vi "数据整合分析.vi"(10 "原始数据库":string[][](table), 11 "Data Result":string[][](table)) -> (3 "原始数据库 2":string[][](table))   [LabVIEW 2015]
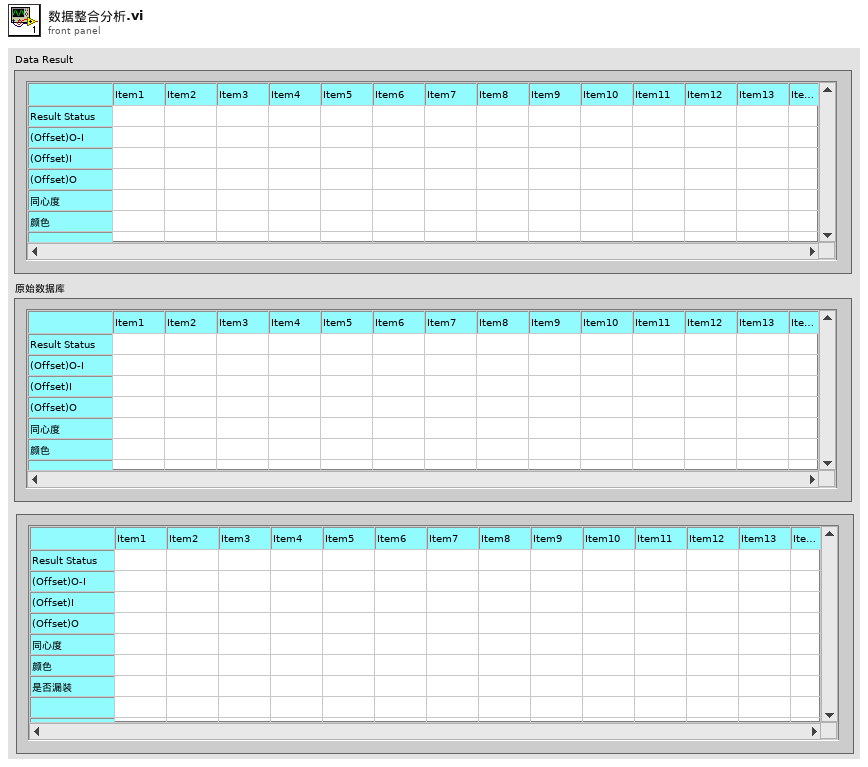
[diagram p1: front panel]
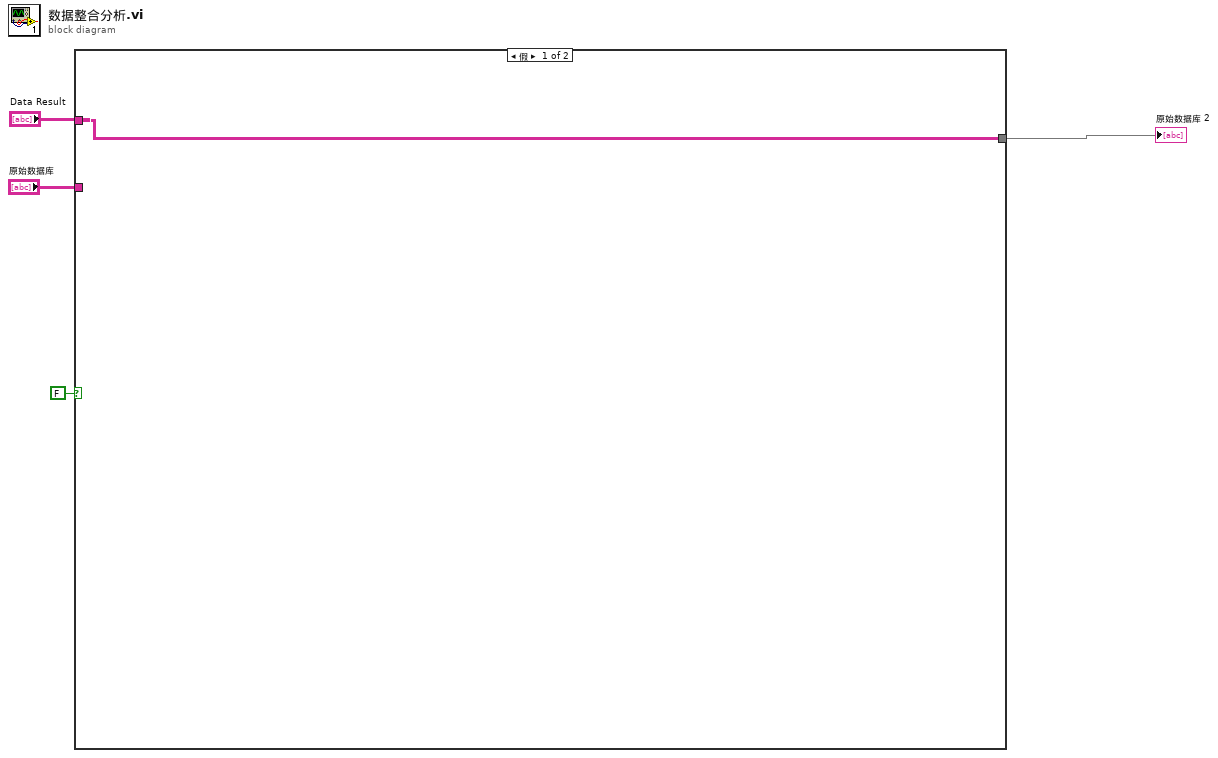
[diagram p0: block diagram]
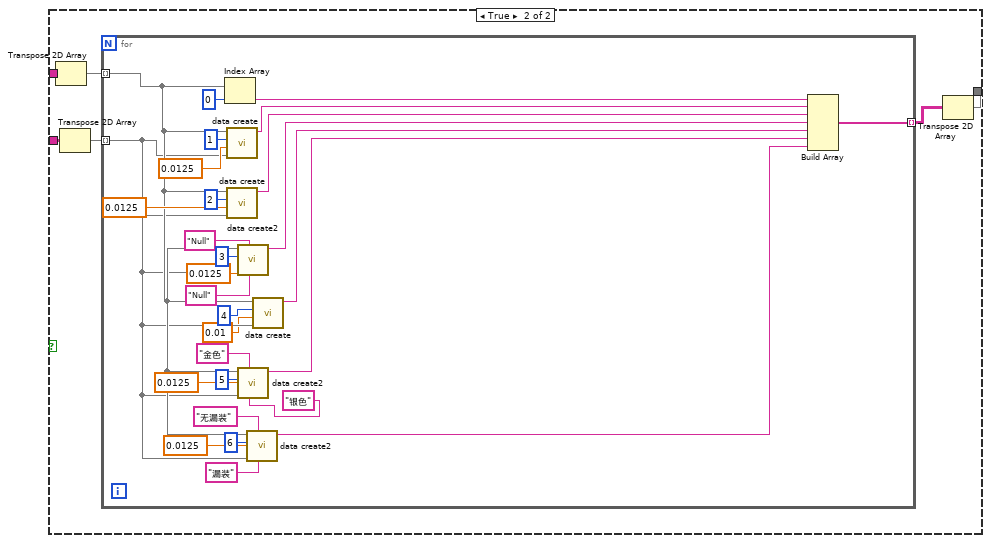
[diagram p2: hidden frame]
diagram:
  n1 = case shown="假" FALSE {
    tunnel: "Data Result" -> [w5 w11]
    tunnel: "原始数据库" -> [_ w9]
    tunnel: [w5 w6] -> w2
    frame False {
    }
    frame True {
      n2 = Transpose 2D Array(2D array=w11) -> (transposed array=w10:string[][])
      n3 = Transpose 2D Array(2D array=w9) -> (transposed array=w8:string[][])
      n4 = for {
        tunnel: w10 -> [w17] mode=indexing
        tunnel: w8 -> [w16] mode=indexing
        tunnel: [w20] -> w7 mode=indexing
        n5 = Index Array(array=w17, index=0 ("索引")) -> (element=w40:string)
        n6 = call "data create.vi"("old"=w16, "y 2"=0.0125, "索引"=1, "new"=w17) -> ("Data"=w36:string)  [unwired: 7 in]
        n7 = call "data create.vi"("old"=w16, "y 2"=0.0125, "索引"=2, "new"=w17) -> ("Data"=w33:string)  [unwired: 7 in]
        n8 = call "data create2.vi"("y 3"="Null", "y"="Null", "old"=w16, "y 2"=0.0125, "索引"=3, "new"=w17) -> ("Data"=w30:string)  [unwired: 5 in]
        n9 = call "data create2.vi"("y 3"="银色" ("y"), "y"="金色", "old"=w16, "y 2"=0.0125, "索引"=5, "new"=w17) -> ("Data"=w25:string)  [unwired: 5 in]
        n10 = call "data create2.vi"("y 3"="漏装", "y"="无漏装", "old"=w16, "y 2"=0.0125, "索引"=6, "new"=w17) -> ("Data"=w21:string)  [unwired: 5 in]
        n11 = call "data create.vi"("old"=w16, "y 2"=0.01, "索引"=4, "new"=w17) -> ("Data"=w13:string)  [unwired: 7 in]
        n12 = Build Array(w40, w36, w33, w30, w13, w25, w21) -> (w20:string[])
      }
      n13 = Transpose 2D Array(2D array=w7) -> (transposed array=w6:string[][])
    }
  }
  "原始数据库 2" <- w2
